vi "Lab08MainVI.vi"() -> ()   [LabVIEW 2022 SP3]
uses:
  VendingMachineControl.ctl
panel:
  out "Current State":T1
  in  "Stop":bool
  out "Message to User":string
  out "Change Returned":dbl format="%.2f"
  in  "Pepsi":bool
  in  "Coke":bool
  out "Coke Display":u16(ring)
  in  "Return Change":bool
  out "Value Deposited":dbl format="%.2f"
  in  "Dime":bool
  in  "Nickel":bool
  in  "Quarter":bool
  # "$0.75"
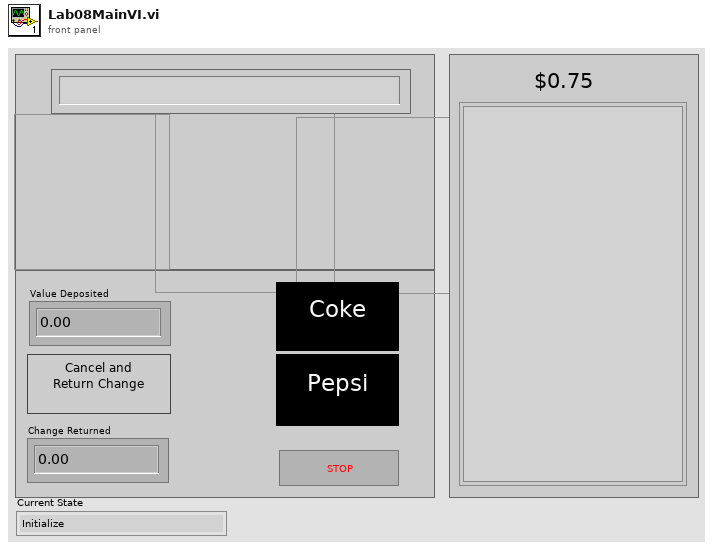
[diagram p1: front panel]
types:
  T1 = typedef "VendingMachineControl.ctl" = enum16{"Initialize", "Stop Check", "Stop", "Wait for UI", "Change Deposited", "Deposit Soda", "Return"}
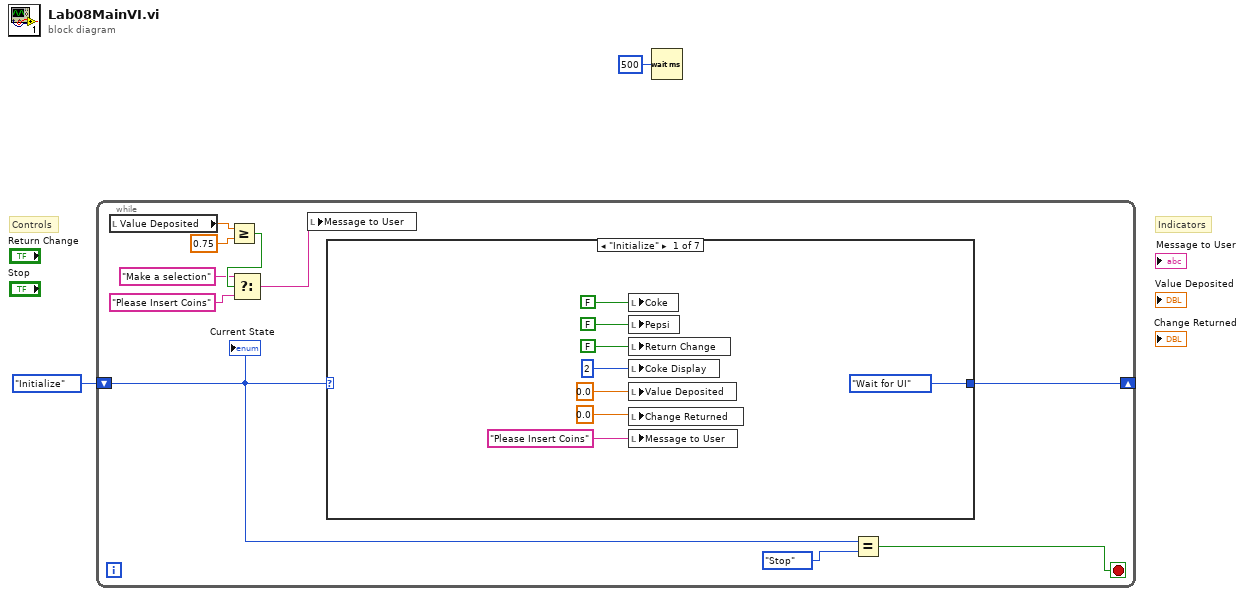
[diagram p0: block diagram]
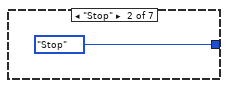
[diagram p2: hidden frame]
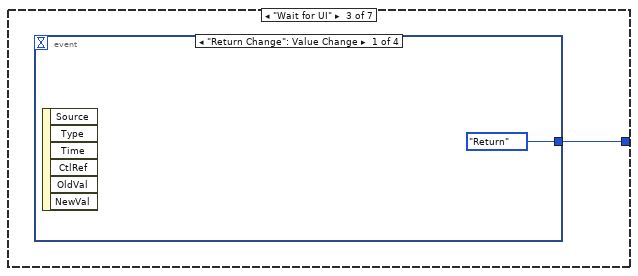
[diagram p3: hidden frame]
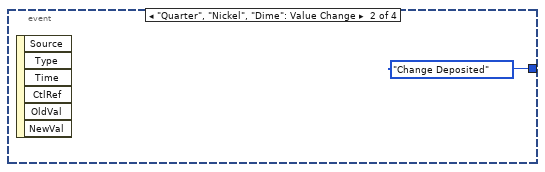
[diagram p4: hidden frame]
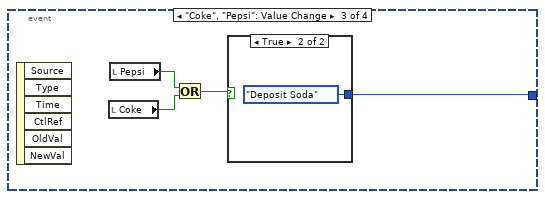
[diagram p5: hidden frame]
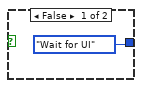
[diagram p6: hidden frame]
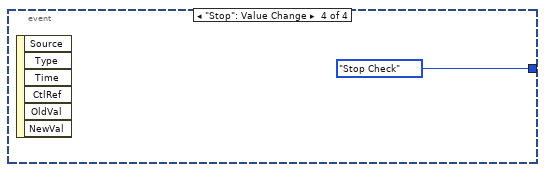
[diagram p7: hidden frame]
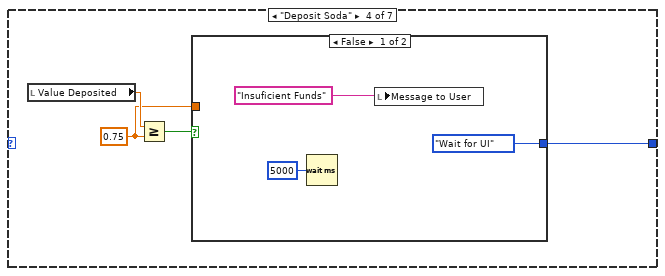
[diagram p8: hidden frame]
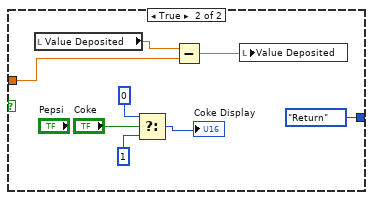
[diagram p9: hidden frame]
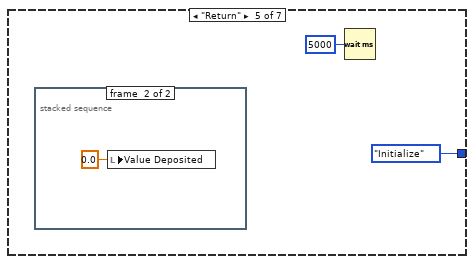
[diagram p10: hidden frame]
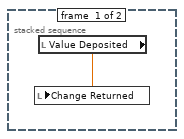
[diagram p11: hidden frame]
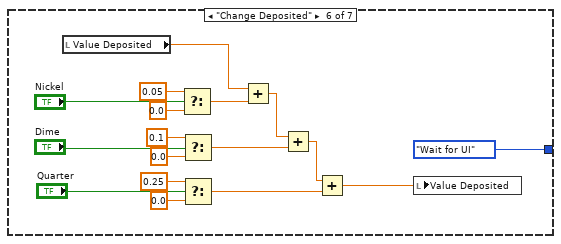
[diagram p12: hidden frame]
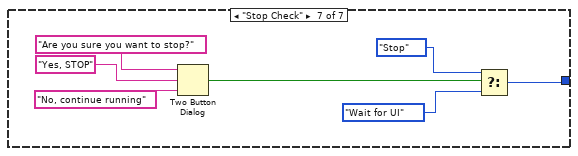
[diagram p13: hidden frame]
diagram:
  # "Indicators"
  # "Controls"
  n1 = while {
    shift-right: [w12] -> _
    shift-left: VendingMachineControl."Initialize" -> [w9]
    stop <- w8 stop-if-true
    n2 = local read "Value Deposited"() -> (w7:dbl)
    n3 = Greater Or Equal?(x=w7, y=0.75) -> (x >= y?=w11:bool)
    n4 = Select(t="Make a selection" ("String"), s=w11, f="Please Insert Coins" ("String")) -> (s? t:f=w5:string)
    n5 = local write "Message to User"(w5) -> ()
    n6 = case shown="\"Initialize\"" w9 {
      tunnel: [VendingMachineControl."Wait for UI" VendingMachineControl."Stop" w22 w35 VendingMachineControl."Initialize" VendingMachineControl."Wait for UI" w68] -> w12
      frame "Initialize" {
        n7 = local write "Coke"(FALSE ("Coke")) -> ()
        n8 = local write "Pepsi"(FALSE ("Pepsi")) -> ()
        n9 = local write "Return Change"(FALSE ("Return Change")) -> ()
        n10 = local write "Coke Display"(u16 2 ("Coke Display")) -> ()
        n11 = local write "Value Deposited"(0.0 ("Numeric 2")) -> ()
        n12 = local write "Change Returned"(0.0 ("Numeric")) -> ()
        n13 = local write "Message to User"("Please Insert Coins" ("String")) -> ()
      }
      frame "Stop" {
      }
      frame "Wait for UI" {
        n14 = event shown="[0] \"Return Change\": Value Change" {
          selector: _ -> [_ _ _ _]
          dyn-events: _ -> [_ _ _ _]
          timeout: _ -> [_ _ _ _]
          tunnel: [VendingMachineControl."Return" VendingMachineControl."Change Deposited" w25 VendingMachineControl."Stop Check"] -> w22
          event "Return Change": Value Change {
            n15 = event-data() -> ()  [unwired: 1 in, 6 out]
          }
          event "Quarter", "Nickel", "Dime": Value Change {
            n16 = event-data() -> ()  [unwired: 1 in, 6 out]
          }
          event "Coke", "Pepsi": Value Change {
            n17 = event-data() -> ()  [unwired: 1 in, 6 out]
            n18 = local read "Coke"() -> (w26:bool)
            n19 = local read "Pepsi"() -> (w27:bool)
            n20 = Or(x=w27, y=w26) -> (x .or. y?=w28:bool)
            n21 = case shown="True" w28 {
              tunnel: [VendingMachineControl."Wait for UI" VendingMachineControl."Deposit Soda"] -> w25
              frame False {
              }
              frame True {
              }
            }
          }
          event "Stop": Value Change {
            n22 = event-data() -> ()  [unwired: 1 in, 6 out]
          }
        }
      }
      frame "Deposit Soda" {
        w32 = 0.75 ("y")
        n23 = local read "Value Deposited"() -> (w34:dbl)
        n24 = Greater Or Equal?(x=w34, y=w32) -> (x >= y?=w33:bool)
        n25 = case shown="False" w33 {
          tunnel: [VendingMachineControl."Wait for UI" VendingMachineControl."Return"] -> w35
          tunnel: w32 -> [_ w45]
          frame False {
            n26 = Wait (ms)(milliseconds to wait=u32 5000) -> ()  [unwired: 1 out]
            n27 = local write "Message to User"("Insuficient Funds" ("String")) -> ()
          }
          frame True {
            n28 = local read "Value Deposited"() -> (w39:dbl)
            n29 = Select(t=0, s="Coke", f=1) -> (s? t:f=→"Coke Display":i32)
            n30 = Subtract(x=w39, y=w45) -> (x-y=w44:dbl)
            n31 = local write "Value Deposited"(w44) -> ()
          }
        }
      }
      frame "Return" {
        n32 = stacked-sequence {
          frame #0 {
            n33 = local read "Value Deposited"() -> (w49:dbl)
            n34 = local write "Change Returned"(w49) -> ()
          }
          frame #1 {
            n35 = local write "Value Deposited"(0.0 ("Value Deposited")) -> ()
          }
        }
        n36 = Wait (ms)(milliseconds to wait=u32 5000) -> ()  [unwired: 1 out]
      }
      frame "Change Deposited" {
        n37 = local read "Value Deposited"() -> (w56:dbl)
        n38 = Select(t=0.05, s="Nickel", f=0.0) -> (s? t:f=w61:dbl)
        n39 = Select(t=0.1, s="Dime", f=0.0) -> (s? t:f=w60:dbl)
        n40 = Select(t=0.25, s="Quarter", f=0.0) -> (s? t:f=w59:dbl)
        n41 = Add(x=w56, y=w61) -> (x+y=w58:dbl)
        n42 = Add(x=w58, y=w60) -> (x+y=w57:dbl)
        n43 = Add(x=w57, y=w59) -> (x+y=w51:dbl)
        n44 = local write "Value Deposited"(w51) -> ()
      }
      frame "Stop Check" {
        n45 = Two Button Dialog(message="Are you sure you want to stop?", 1:"No, continue running" ("Center Button Text (\"No\")"), 2:"Yes, STOP" ("Left Button Text (\"Yes\")")) -> (T button?=w70:bool)
        n46 = Select(t=VendingMachineControl."Stop", s=w70, f=VendingMachineControl."Wait for UI") -> (s? t:f=w68:T1)
      }
    }
    n47 = Equal?(x=w9, y=VendingMachineControl."Stop") -> (x = y?=w8:bool)
    "Current State" <- w9
  }
  n48 = Wait (ms)(milliseconds to wait=u32 500) -> ()  [unwired: 1 out]
